vi "DT3120_BArrayToInfoStruct.vi"(10 "iCount":i32, 11 "lpDevList":u8[](array[numeric])=[52, 0, 0, 0, 3, 0, 0, 0, 128, 128, 0, 0, 68, 84, 51, 49, 50, 48, 75, 45, 49, 0, 0, 0, 0, 0, 0, 0, 0, 0, 0, 0, 68, 116, 51, 49, 50, 48, 75, 0, 0, 0, 0, 0, 0, 0, 0, 0, 0, 0, 0, 0, 0, 0, 0, 0, 0, 0, 0, 0, 0, 0, 0, 0, 0, 0, 0, 0, 0, 0, 0, 0, 0, 0, 0, 0, 0, 0, 0, 0, 0, 0, 0, 0, 0, 0, 0, 0, 0, 0, 0, 0, 0, 0, 0, 0, 0, 0, 0, 0, 0, 0, 0, 0, 0, 0, 0, 0, 0, 0, 0, 0, 0, 0, 0, 0, 0, 0, 0, 0, 0, 0, 0, 0, 0, 0, 0, 0, 0, 0, 0, 0, 0, 0, 0, 0, 0, 0, 0, 0, 0, 0, 0, 0, 0, 0, 0, 0, 0, 0, 0, 0, 0, 0, 0, 0, 0, 0, 0, 0, 0, 0, 0, 0, 0, 0, 0, 0, 0, 0, 0, 0, 0, 0, 0, 0, 0, 0, 0, 0, 0, 0, 0, 0, 0, 0, 0, 0, 0, 0, 0, 0, 0, 0, 0, 0, 0, 0, 0, 0, 0, 0, 0, 0, 0, 0, 0, 0, 0, 0, 0, 0, 0, 0, 0, 0, 0, 0, 0, 0, 0, 0, 0, 0, 0, 0, 0, 0, 0, 0, 0, 0, 0, 0, 0, 0, 0, 0, 0, 0, 0, 0, 0, 0, 0, 0, 0, 0, 0, 0, 0, 0, 0, 0, 0, 0, 0, 0, 0, 0, 0, 0, 0, 0, 0, 0, 0, 0, 0, 0, 0, 0, 0, 0, 0, 0, 0, 0, 0, 0, 0, 0, 0, 0, 0, 0, 0, 0, 0, 0, 0, 0, 0, 0, 0, 0, 0, 0, 0, 0, 0, 0, 0, 0, 0, 0, 0, 0, 0, 0, 0, 0, 0, 0, 0, 0, 0, 0, 0, 0, 0, 0, 0, 0, 0, 0, 0, 0, 0, 0, 0, 0, 0, 0, 0, 0, 0, 0, 0, 0, 0, 0, 0, 0, 0, 0, 0, 0, 0, 0, 0, 0, 0, 0, 0, 0, 0, 0, 0, 0, 0, 0, 0, 0, 0, 0, 0, 0, 0, 0, 0, 0, 0, 0, 0, 0, 0, 0, 0, 0, 0, 0, 0, 0, 0, 0, 0, 0, 0, 0, 0, 0, 0, 0, 0, 0, 0, 0, 0, 0, 0, 0, 0, 0, 0, 0, 0, 0, 0, 0, 0, 0, 0, 0, 0, 0, 0, 0, 0, 0, 0, 0, 0, 0, 0, 0, 0, 0, 0, 0, 0, 0, 0, 0, 0, 0, 0, 0, 0, 0, 0, 0, 0, 0, 0, 0, 0, 0, 0, 0, 0, 0, 0, 0, 0, 0, 0, 0, 0, 0, 0, 0, 0, 0, 0, 0, 0, 0, 0, 0, 0, 0, 0, 0, 0, 0, 0, 0, 0, 0, 0, 0, 0, 0, 0, 0, 0, 0, 0, 0, 0, 0, 0, 0, 0, 0, 0, 0, 0, 0, 0, 0, 0, 0, 0, 0, 0, 0, 0, 0, 0, 0, 0, 0, 0, 0, 0, 0, 0, 0, 0, 0, 0, 0, 0, 0, 0, 0, 0, 0, 0, 0, 0, 0, 0, 0, 0, 0, 0, 0, 0, 0, 0, 0, 0, 0, 0, 0, 0, 0, 0, 0, 0, 0, 0, 0, 0, 0, 0, 0, 0, 0, 0, 0, 0, 0, 0, 0, 0, 0, 0, 0, 0, 0, 0, 0, 0, 0, 0, 0, 0, 0, 0, 0, 0, 0, 0, 0, 0, 0, 0, 0, 0, 0, 0, 0, 0, 0, 0, 0, 0, 0, 0, 0, 0, 0, 0, 0, 0, 0, 0, 0, 0, 0, 0, 0, 0, 0, 0, 0, 0, 0, 0, 0, 0, 0, 0, 0, 0, 0, 0, 0, 0, 0, 0, 0, 0, 0, 0, 0, 0, 0, 0, 0, 0, 0, 0, 0, 0, 0, 0, 0, 0, 0, 0, 0, 0, 0, 0, 0, 0, 0, 0, 0, 0, 0, 0, 0, 0, 0, 0, 0, 0, 0, 0, 0, 0, 0, 0, 0, 0, 0, 0, 0, 0, 0, 0, 0, 0, 0, 0, 0, 0, 0, 0, 0, 0, 0, 0, 0, 0, 0, 0, 0, 0, 0, 0, 0, 0, 0, 0, 0, 0, 0, 0, 0, 0, 0, 0, 0, 0, 0, 0, 0, 0, 0, 0, 0, 0, 0, 0, 0, 0, 0, 0, 0, 0, 0, 0, 0, 0, 0, 0, 0, 0, 0, 0, 0, 0, 0, 0, 0, 0, 0, 0, 0, 0, 0, 0, 0, 0, 0, 0, 0, 0, 0, 0, 0, 0, 0, 0, 0, 0, 0, 0, 0, 0, 0, 0, 0, 0, 0, 0, 0, 0, 0, 0, 0, 0, 0, 0, 0, 0, 0, 0, 0, 0, 0, 0, 0, 0, 0, 0, 0, 0, 0, 0, 0, 0, 0, 0, 0, 0, 0, 0, 0, 0, 0, 0, 0, 0, 0, 0, 0, 0, 0, 0, 0, 0, 0, 0, 0, 0, 0, 0, 0, 0, 0, 0, 0, 0, 0, 0, 0, 0, 0, 0, 0, 0, 0, 0, 0, 0, 0, 0, 0, 0, 0, 0, 0, 0, 0, 0, 0, 0, 0, 0, 0, 0, 0, 0, 0, 0, 0, 0, 0, 0, 0, 0, 0, 0, 0, 0, 0, 0, 0, 0, 0, 0, 0, 0, 0, 0, 0, 0, 0, 0, 0, 0, 0, 0, 0, 0, 0, 0, 0, 0, 0, 0, 0, 0, 0, 0, 0, 0, 0, 0, 0, 0, 0, 0, 0, 0, 0, 0, 0, 0, 0, 0, 0, 0, 0, 0, 0, 0, 0, 0, 0, 0, 0, 0, 0, 0, 0, 0, 0, 0, 0, 0, 0, 0, 0, 0, 0, 0, 0, 0, 0, 0, 0, 0, 0, 0, 0, 0, 0, 0, 0, 0, 0, 0, 0, 0, 0, 0, 0, 0, 0, 0, 0, 0, 0, 0, 0, 0, 0, 0, 0, 0, 0, 0, 0, 0, 0, 0, 0, 0, 0, 0, 0, 0, 0, 0, 0, 0, 0, 0, 0, 0, 0, 0, 0, 0, 0, 0, 0, 0, 0, 0, 0, 0, 0, 0, 0]) -> (2 "Alias List":string[](array[string]), 3 "Device List":T1(array[cluster]))   [LabVIEW 2013]
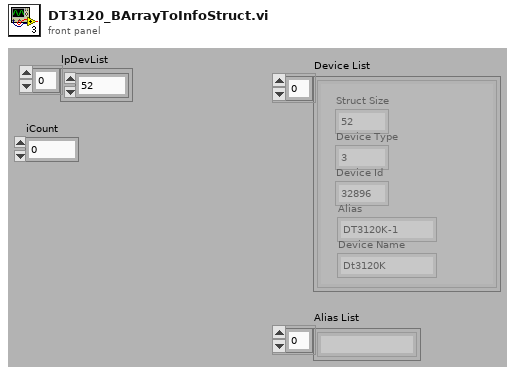
[diagram p1: front panel]
types:
  T1 = cluster{"Struct Size":u32, "Device Type":u32, "Device Id":u32, "Alias":string, "Device Name":string}[]
  T2 = cluster{u32, u32, u32, "string":string, "string":string}
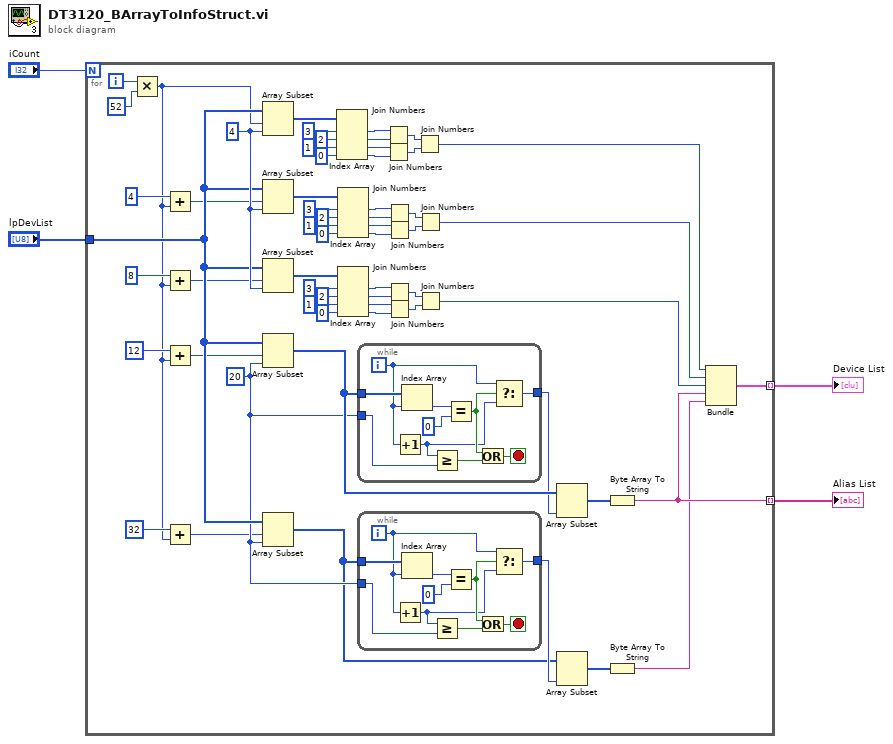
[diagram p0: block diagram]
diagram:
  n1 = for {
    N: "iCount" -> [_]
    tunnel: "lpDevList" -> [w62]
    tunnel: [w7] -> w2 mode=indexing
    tunnel: [w5] -> w1 mode=indexing
    i -> [w21]
    w24 = 20 ("length")
    w63 = 4 ("length")
    n2 = Multiply(x=w21, y=52 ("ulListSize")) -> (x*y=w11:i32)
    n3 = Add(x=4 ("index"), y=w11) -> (x+y=w18:i32)
    n4 = Add(x=8 ("index"), y=w11) -> (x+y=w17:i32)
    n5 = Add(x=12 ("index"), y=w11) -> (x+y=w15:i32)
    n6 = Add(x=32 ("index"), y=w11) -> (x+y=w13:i32)
    n7 = Array Subset(array=w62, index=w11, length=w63) -> (w58:u8[])
    n8 = Array Subset(array=w62, index=w18, length=w63) -> (w40:u8[])
    n9 = Array Subset(array=w62, index=w17, length=w63) -> (w29:u8[])
    n10 = Array Subset(array=w62, index=w15, length=w24) -> (w28:u8[])
    n11 = Array Subset(array=w62, index=w13, length=w24) -> (w23:u8[])
    n12 = Index Array(array=w58, index #1=3 ("index"), index #2=2 ("index"), index #3=1 ("index"), index #4=0 ("index")) -> (element #1=w57:u8, element #2=w56:u8, element #3=w55:u8, element #4=w54:u8)
    n13 = Index Array(array=w40, index #1=3 ("index"), index #2=2 ("index"), index #3=1 ("index"), index #4=0 ("index")) -> (element #1=w47:u8, element #2=w46:u8, element #3=w45:u8, element #4=w44:u8)
    n14 = Index Array(array=w29, index #1=3 ("index"), index #2=2 ("index"), index #3=1 ("index"), index #4=0 ("index")) -> (element #1=w36:u8, element #2=w35:u8, element #3=w34:u8, element #4=w33:u8)
    n15 = while {
      tunnel: w28 -> [w83]
      tunnel: w24 -> [w78]
      tunnel: [w74] -> w27
      i -> [w76]
      stop <- w80 stop-if-true
      n16 = Increment(x=w76) -> (x+1=w75:i32)
      n17 = Index Array(array=w83, index=w76) -> (element=w82:u8)
      n18 = Greater Or Equal?(x=w75, y=w78) -> (x >= y?=w79:bool)
      n19 = Equal?(x=w82, y=u8 0) -> (x = y?=w77:bool)
      n20 = Or(x=w77, y=w79) -> (x .or. y?=w80:bool)
      n21 = Select(t=w76, s=w77, f=w75) -> (s? t:f=w74:i32)
    }
    n22 = while {
      tunnel: w23 -> [w73]
      tunnel: w24 -> [w68]
      tunnel: [w64] -> w25
      i -> [w66]
      stop <- w70 stop-if-true
      n23 = Increment(x=w66) -> (x+1=w65:i32)
      n24 = Index Array(array=w73, index=w66) -> (element=w72:u8)
      n25 = Greater Or Equal?(x=w65, y=w68) -> (x >= y?=w69:bool)
      n26 = Equal?(x=w72, y=u8 0) -> (x = y?=w67:bool)
      n27 = Or(x=w67, y=w69) -> (x .or. y?=w70:bool)
      n28 = Select(t=w66, s=w67, f=w65) -> (s? t:f=w64:i32)
    }
    n29 = Join Numbers(hi=w57, lo=w56) -> ((hi.lo)=w53:u16)
    n30 = Join Numbers(hi=w55, lo=w54) -> ((hi.lo)=w52:u16)
    n31 = Join Numbers(hi=w47, lo=w46) -> ((hi.lo)=w43:u16)
    n32 = Join Numbers(hi=w45, lo=w44) -> ((hi.lo)=w42:u16)
    n33 = Join Numbers(hi=w36, lo=w35) -> ((hi.lo)=w32:u16)
    n34 = Join Numbers(hi=w34, lo=w33) -> ((hi.lo)=w31:u16)
    n35 = Join Numbers(hi=w53, lo=w52) -> ((hi.lo)=w10:u32)
    n36 = Join Numbers(hi=w43, lo=w42) -> ((hi.lo)=w8:u32)
    n37 = Join Numbers(hi=w32, lo=w31) -> ((hi.lo)=w9:u32)
    n38 = Array Subset(array=w28, length=w27) -> (w26:u8[])  [unwired: 1 in]
    n39 = Array Subset(array=w23, length=w25) -> (w22:u8[])  [unwired: 1 in]
    n40 = Byte Array To String(unsigned byte array=w26) -> (string=w7:string)
    n41 = Byte Array To String(unsigned byte array=w22) -> (string=w6:string)
    n42 = Bundle(w10, w8, w9, "string"=w7, "string"=w6) -> (w5:T2)  [unwired: 1 out]
  }
  "Alias List" <- w2
  "Device List" <- w1
